vi "Function code mismatch error.vi"(8 "error in (no error)":errorcluster) -> (0 "error out":errorcluster)   [LabVIEW 2021, in "Master Function Definition.lvclass"]
uses:
  Master Function Definition.lvclass
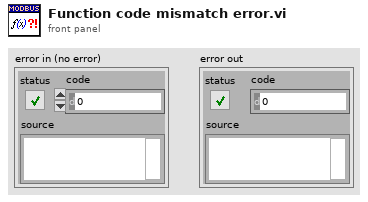
[diagram p1: front panel]
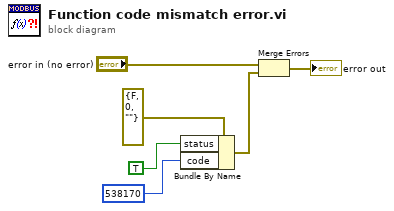
[diagram p0: block diagram]
diagram:
  n1 = Bundle By Name(cluster=errorcluster {"status"=FALSE, "code"=0, "source"=""} ("error constant"), "status"=TRUE, "code"=538170) -> (w3:errorcluster)
  n2 = Merge Errors("error in (no error)", w3) -> (→"error out":errorcluster)
